vi "GetPathToNetworkImpairPlugin.vi"(8 "ErrorArray In":errorcluster[](array[cluster]), 11 "Bus.lvclass In":refnum<class "Bus.lvclass">) -> (0 "ErrorArray Out":errorcluster[](array[cluster]), 2 "NetImpPluginINIFilePath":path, 3 "Bus.lvclass Out":refnum<class "Bus.lvclass">)   [LabVIEW 2014]
uses:
  <userlib>/NIST/NISTErrorLib/NISTErrorLib.lvlib
  <vilib>/Utility/error.llb/Error Cluster From Error Code.vi
  <vilib>/ErrorRing/Error Ring.xnode
  NetworkImpairment/NetworkImpairmentModule/NetworkImpairmentModule.lvlib
  NetworkImpairment/NetworkImpairmentModule/PublicAPI/Arguments/Requests/clLoadPlugin.ctl
  Bus.lvclass
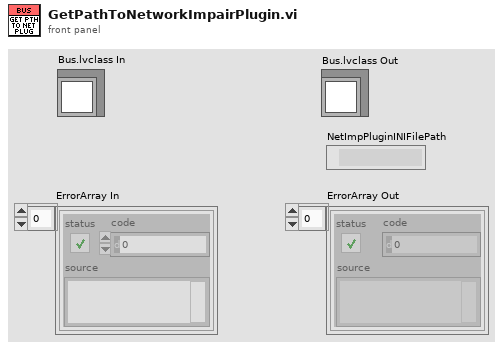
[diagram p1: front panel]
types:
  T1 = typedef "NetworkImpairmentModule.lvlib/clBroadcastEvents.ctl" = cluster{"DidInit":refnum<user-event>, "StatusUpdate":refnum<user-event>, "ErrorReport":refnum<user-event>, "DidStop":refnum<user-event>, "ReadNetImpParams":refnum<user-event>, "ReadLossThreshold":refnum<user-event>, "GetNetworkTime":refnum<user-event>, "GetPktLoss":refnum<user-event>, "ReadPathToPlugin":refnum<user-event>}
  T2 = typedef "NetworkImpairmentModule.lvlib/clLoadPlugin.ctl" = cluster{"PathToPlugin":path}
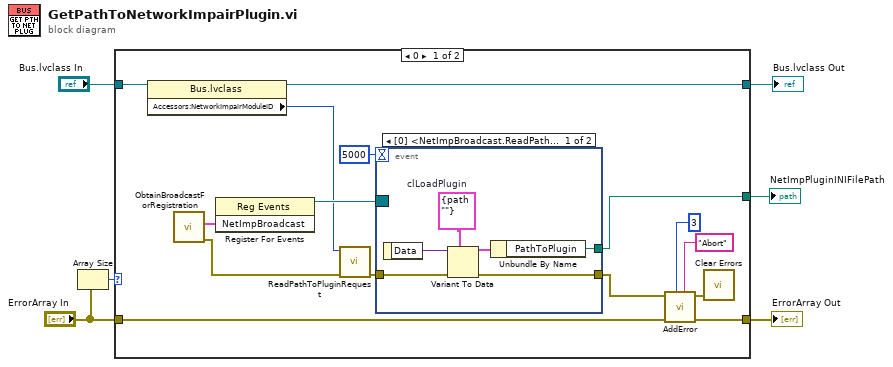
[diagram p0: block diagram]
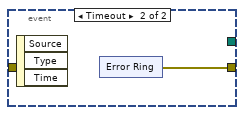
[diagram p2: hidden frame]
diagram:
  n1 = Array Size(array="ErrorArray In") -> (size(s)=w5:i32)
  n2 = case shown="0" w5 {
    tunnel: "ErrorArray In" -> [w21 w35]
    tunnel: [w20 w35] -> w6
    tunnel: "Bus.lvclass In" -> [w16 w34]
    tunnel: [w10 w34] -> w2
    tunnel: [w9 _] -> w1
    frame 0 {
      n3 = property class="Bus.lvclass"(reference=w16) -> (reference out=w10:refnum<class "Bus.lvclass">, "Accessors:NetworkImpairModuleID"=w11:i32)  [unwired: 1 in, 1 out]
      n4 = call "ObtainBroadcastForRegistration.vi"() -> ("error out"=w13:errorcluster, "NetImpBroadcast"=w15:T1)  [unwired: 10 in]
      n5 = register-events(w15) -> (reference out=w14:refnum<event-registration>)  [unwired: 2 in, 1 out]
      n6 = call "ReadPathToPluginRequest.vi"("error in (no error)"=w13, "ModuleID"=w11) -> ("error out"=w12:errorcluster)  [unwired: 9 in]
      n7 = event shown="[0] <NetImpBroadcast.ReadPathToPlugin>: User Event" {
        selector: w14 -> [_ _]
        dyn-events: _ -> [_ _]
        timeout: 5000 -> [_ _]
        tunnel: w12 -> [w26 _]
        tunnel: [w23 _] -> w9
        tunnel: [w22 w28] -> w8
        event User Event {
          w25 = T2 {"PathToPlugin"=path ""}  # clLoadPlugin
          n8 = event-data() -> ("Data"=w27:variant)  [unwired: 1 in]
          n9 = Variant To Data(error in=w26, type=w25, Variant=w27) -> (data=w24:T2, error out=w22:errorcluster)
          n10 = Unbundle By Name(w24) -> ("PathToPlugin"=w23:path)
        }
        event Timeout {
          n11 = event-data() -> ()  [unwired: 1 in, 3 out]
          n12 = xnode "Error Ring"() -> ("error out"=w28:errorcluster)
        }
      }
      n13 = call <userlib>:"AddError.vi"("Severity"="Abort" ("String"), "Priority"=u8 3, "ErrorArray"=w21, "error in (no error)"=w8) -> ("ErrorArray"=w20:errorcluster[], "error out"=w19:errorcluster)  [unwired: 6 in]
      n14 = call <vilib>:"Clear Errors.vi"("error in (no error)"=w19) -> ()  [unwired: 5 in, 2 out]
    }
    frame 1, Default {
    }
  }
  "ErrorArray Out" <- w6
  "Bus.lvclass Out" <- w2
  "NetImpPluginINIFilePath" <- w1
